vi "Reset Button Color.vi"(8 "error in (no error)":errorcluster, 11 "Control in":refnum<vi>) -> (0 "error out":errorcluster)   [LabVIEW 2011]
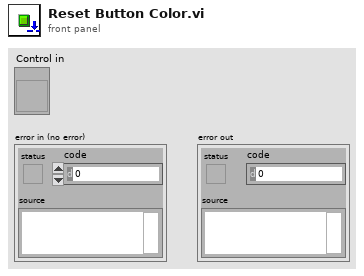
[diagram p1: front panel]
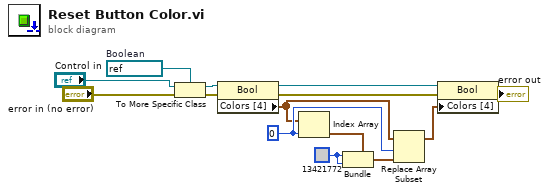
[diagram p0: block diagram]
diagram:
  w10 = 0 ("index")
  w4 = u32 13421772
  w3 = refnum<vi> refnum  # Boolean
  n1 = To More Specific Class(target class=w3, reference="Control in", error in="error in (no error)") -> (specific class reference=w12:refnum<vi>, error out=w13:errorcluster)
  n2 = property on="Property Node" class="Bool"(reference=w12, error in=w13) -> (reference out=w6:refnum<vi>, error out=w5:errorcluster, "Colors [4]"=w8:cluster{u32, u32}[])
  n3 = Index Array(array=w8, index=w10) -> (element=w7:cluster{u32, u32})
  n4 = Bundle(cluster=w7, w4, w4) -> (w9:cluster{u32, u32})
  n5 = Replace Array Subset(array=w8, new element=w9, index=w10) -> (w11:cluster{u32, u32}[])
  n6 = property on="Property Node" class="Bool"(reference=w6, error in=w5, "Colors [4]"=w11) -> (error out=→"error out":errorcluster)  [unwired: 1 out]
